vi "TeleopGyro.vi"() -> ()   [LabVIEW 2015]
uses:
  <vilib>/Rock Robotics/Network Tables/NT Write Number.vi
panel:
  out "Calibrated?":bool
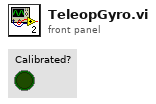
[diagram p1: front panel]
types:
  T1 = typedef "WPI_GyroDevRef.ctl" = cluster{"DevStatus":errorcluster, "Analog Channel":T2, "Offset":dbl, "Gain (VoltsPerDegree/Second)":dbl, "Gyro Type":enum16{"Analog", "XRS450"}, "Handle":i32, "SPI Bus":T3, "Device Found":bool, "Sample Rate":dbl, "Calibrate On Open":bool}
  T2 = typedef "FPGA_AIChannel.ctl" = enum8{"AI 0", "AI 1", "AI 2", "AI 3", "AI MXP 0", "AI MXP 1", "AI MXP 2", "AI MXP 3", "Invalid"}
  T3 = typedef "spi_bus.ctl" = enum16{"SPI On-Board, CS0", "SPI On-Board, CS1", "SPI On-Board, CS2", "SPI On-Board, CS3", "SPI MXP", "Invalid"}
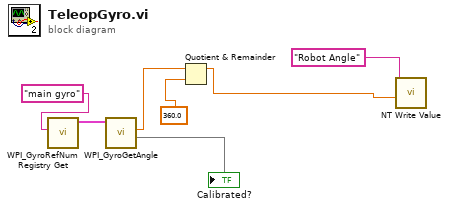
[diagram p0: block diagram]
diagram:
  n1 = call <vilib>:"WPI_GyroRefNum Registry Get.vi"("refnum name"="main gyro") -> ("GyroDevRef"=w6:T1)  [unwired: 9 in, 1 out]
  n2 = call <vilib>:"WPI_GyroGetAngle.vi"("GyroDevRef"=w6) -> ("Angle"=w4:dbl, 4:→"Calibrated?")  [unwired: 6 in, 3 out]
  n3 = Quotient & Remainder(x=w4, y=360.0) -> (x-y*floor(x/y)=w1:dbl)  [unwired: 1 out]
  n4 = call-poly <vilib>:"NT Write Value.vi"("Numeric"=w1, "Name"="Robot Angle") -> ()  [unwired: 9 in, 1 out]
